vi "LS Data Global.vi"(0 "Recording In":bool, 2 "Mode":T2(ring), 5 "Initial LS Data In":T1={"Total Cycles"=[0, 0, 0, 0, 0, 0, 0, 0, 0, 0, 0, 0], "Steps"=[0, 0, 0, 0, 0, 0, 0, 0, 0, 0, 0, 0], "Anomalies Total"=[0, 0, 0, 0, 0, 0, 0, 0, 0, 0, 0, 0], "Cycles"=[0, 0, 0, 0, 0, 0, 0, 0, 0, 0, 0, 0], "Anomalies/Cycle"=[0, 0, 0, 0, 0, 0, 0, 0, 0, 0, 0, 0], "Anomalies (Last Cycle)"=[0, 0, 0, 0, 0, 0, 0, 0, 0, 0, 0, 0], "Opens"=[0, 0, 0, 0, 0, 0, 0, 0, 0, 0, 0, 0]} {"Opens" format="%#.0f"; "Anomalies (Last Cycle)" format="%#.0f"; "Anomalies/Cycle" format="%#.0f"; "Cycles" format="%#.0f"; "Anomalies Total" format="%#.0f"; "Steps" format="%#.0f"; "Total Cycles" format="%#.0f"}, 7 "LS Cluster In":T3, 11 "Transferring In":bool) -> (4 "Recording Out":bool, 6 "Initial LS Data Out":T1 {"Opens" format="%#.0f"; "Anomalies (Last Cycle)" format="%#.0f"; "Anomalies/Cycle" format="%#.0f"; "Cycles" format="%#.0f"; "Anomalies Total" format="%#.0f"; "Steps" format="%#.0f"; "Total Cycles" format="%#.0f"}, 8 "LS Cluster Out":T3, 15 "Transferring Out":bool)   [LabVIEW 2018]
uses:
  Type Defs/LS Data.ctl
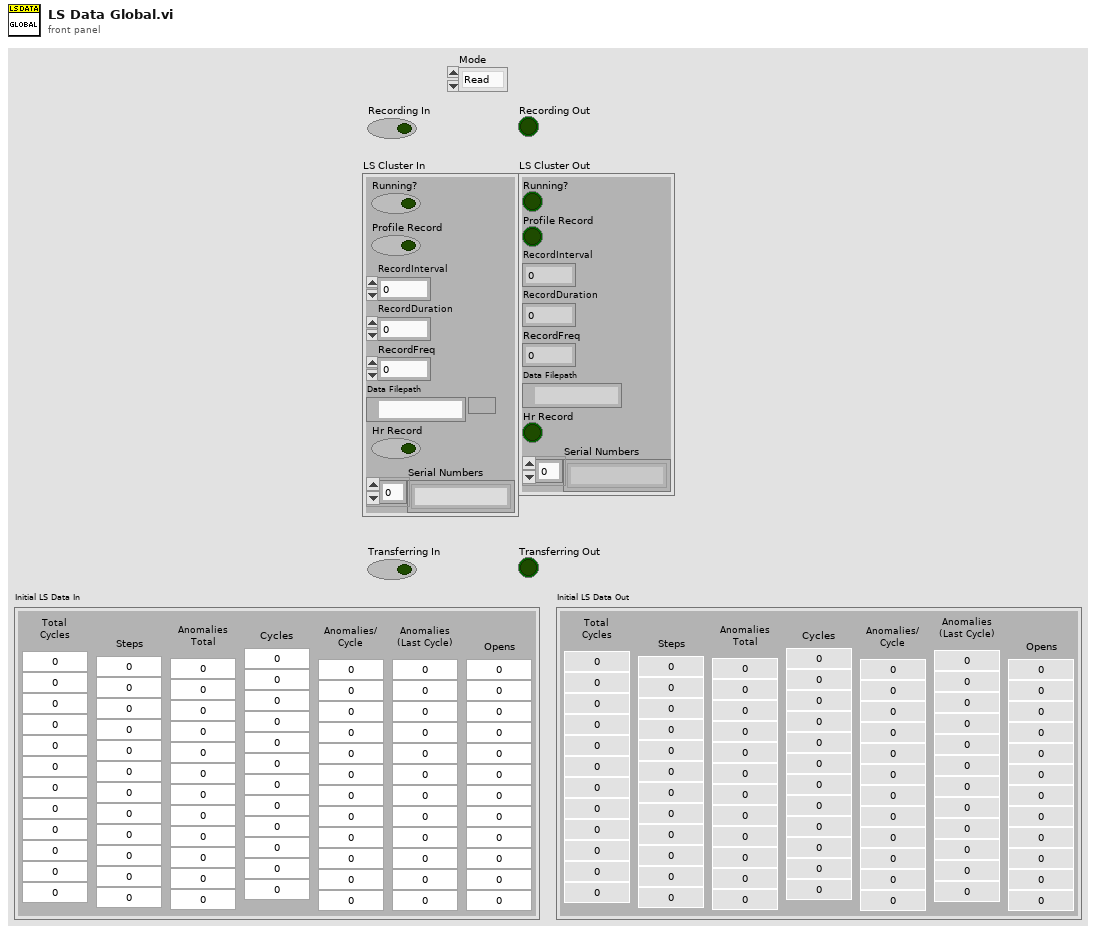
[diagram p1: front panel]
types:
  T1 = typedef "LS Data.ctl" = cluster{"Total Cycles":u32[], "Steps":u32[], "Anomalies Total":i32[], "Cycles":u32[], "Anomalies/Cycle":i32[], "Anomalies (Last Cycle)":i32[], "Opens":i32[]}
  T2 = enum16{"Read", "Engine Writes", "Main Writes", "Write Anomalies", "Write Init Data"}
  T3 = cluster{"Running?":bool, "Profile Record":bool, "RecordInterval":i32, "RecordDuration":i32, "RecordFreq":i32, "Data Filepath":path, "Hr Record":bool, "Serial Numbers":string[]}
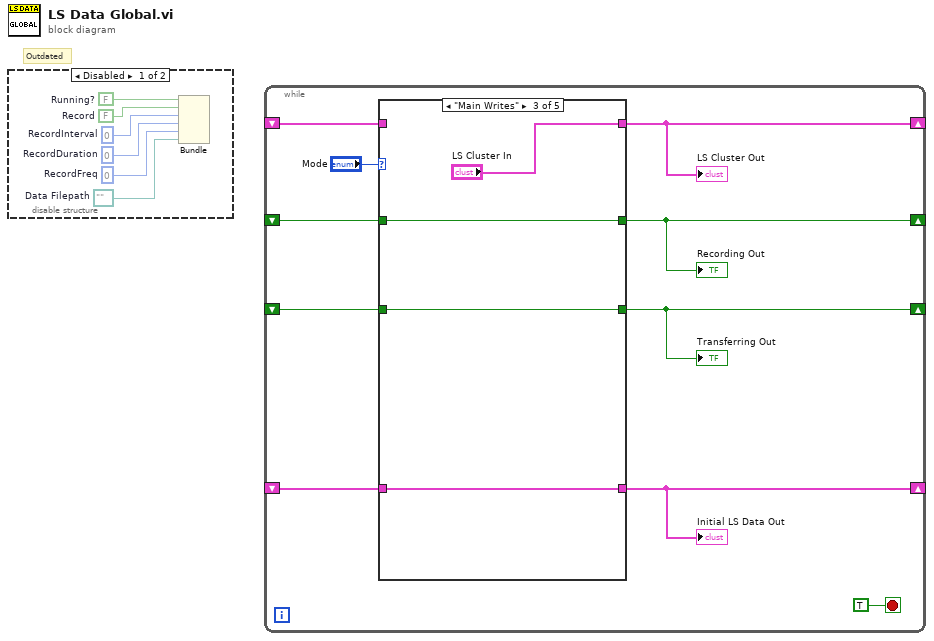
[diagram p0: block diagram]
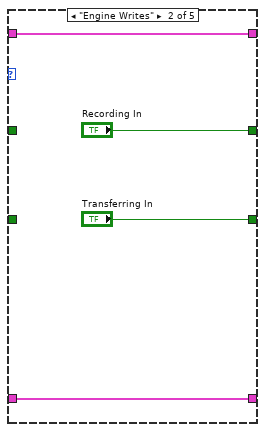
[diagram p4: hidden frame]
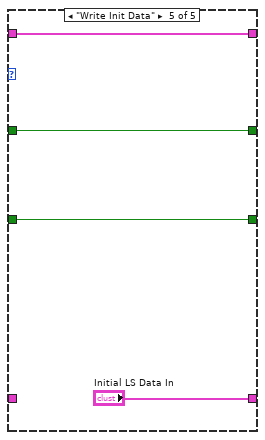
[diagram p6: hidden frame]
diagram:
  # "Outdated"
  n1 = disable-structure shown="Disabled" {
    frame Disabled {
      w1 = path ""  # Data Filepath
      w2 = 0  # RecordFreq
      w3 = 0  # RecordDuration
      w4 = 0  # RecordInterval
      w5 = FALSE  # Record
      w6 = FALSE  # Running?
      n2 = Bundle("Running?"=w6, "Record"=w5, "RecordInterval"=w4, "RecordDuration"=w3, "RecordFreq"=w2, "Data Filepath"=w1) -> ()  [unwired: 1 in, 1 out]
    }
    frame Enabled {
    }
  }
  n3 = while {
    shift-right: [w14] -> _
    shift-left: _ -> [w15]
    shift-right: [w11] -> _
    shift-left: _ -> [w12]
    shift-right: [w9] -> _
    shift-left: _ -> [w10]
    shift-right: [w7] -> _
    shift-left: _ -> [w8]
    stop <- TRUE stop-if-true
    n4 = case shown="\"Main Writes\"" "Mode" {
      tunnel: w15 -> [w20 w24 _ w30 w33]
      tunnel: [w20 w24 "LS Cluster In" w30 w33] -> w14
      tunnel: w12 -> [w19 _ w27 w31 w34]
      tunnel: [w19 "Recording In" w27 w31 w34] -> w11
      tunnel: [w18 "Transferring In" w26 w32 w35] -> w9
      tunnel: w10 -> [w18 _ w26 w32 w35]
      tunnel: [w17 w21 w25 w29 "Initial LS Data In"] -> w7
      tunnel: w8 -> [w17 w21 w25 w29 _]
      frame "Read", Default {
      }
      frame "Engine Writes" {
      }
      frame "Main Writes" {
      }
      frame "Write Anomalies" {
      }
      frame "Write Init Data" {
      }
    }
    "LS Cluster Out" <- w14
    "Recording Out" <- w11
    "Transferring Out" <- w9
    "Initial LS Data Out" <- w7
  }
